vi "swmm_close.vi"(3 "error in (no error)":errorcluster, 5 "Success msg?":bool) -> (0 "error out":errorcluster)   [LabVIEW 2014]
uses:
  swmm5.dll
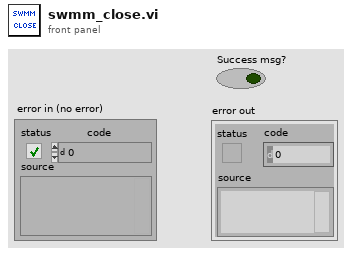
[diagram p1: front panel]
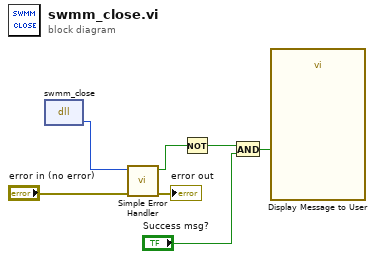
[diagram p0: block diagram]
diagram:
  n1 = dll-call lib="PTH2zabs CUsers\nandres riañoDropboxProyecto AguasSoftwareMatSWMMMatSWMM 5.1.009LabVIEW modulex64\tswmm5.dll" fn="swmm_close"() -> ("return type"=w3:i32)  [unwired: 3 in, 2 out]
  n2 = call <vilib>:"Simple Error Handler.vi"("error code (no error:0)"=w3, "error in (no error)"="error in (no error)") -> ("error?"=w2:bool, "error out"=→"error out":errorcluster)  [unwired: 3 in, 3 out]
  n3 = Not(x=w2) -> (.not. x?=w1:bool)
  n4 = And(x=w1, y="Success msg?") -> (x .and. y?=w4:bool)
  n5 = call "Display Message to User"("Enable"=w4) -> ()  [unwired: 9 in, 2 out]
